vi "Move.vi"(8 "error in (no error)":errorcluster caption="错误输入（无错误）", 10 "samples per channel":i32=1000 caption="脉冲数", 11 "Hardware Resources in":T1 caption="硬件资源输入") -> (0 "error out":errorcluster caption="错误输出", 3 "Hardware Resources out":T1 caption="硬件资源输出")   [LabVIEW 2015, in "Motor Control.lvlib"]
doc: "初始化硬件引用。"
uses:
  Motor Control.lvlib
  Hardware Configuration.ctl
  <vilib>/DAQmx/create/channels.llb/DAQmx Create Channel (CO-Pulse Generation-Frequency).vi
  <vilib>/DAQmx/configure/timing.llb/DAQmx Timing (Implicit).vi
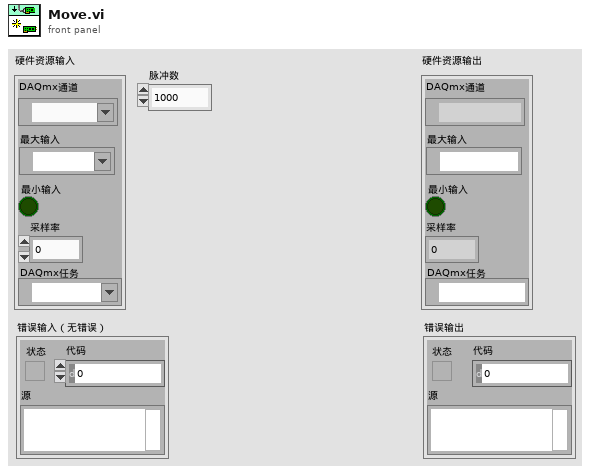
[diagram p1: front panel]
types:
  T1 = typedef "Motor Control.lvlib/Hardware Configuration.ctl" = cluster{"counter":tag, "方向端口":tag, "当前方向":bool, "频率":dbl, "DAQmx Task":refnum<k21>}
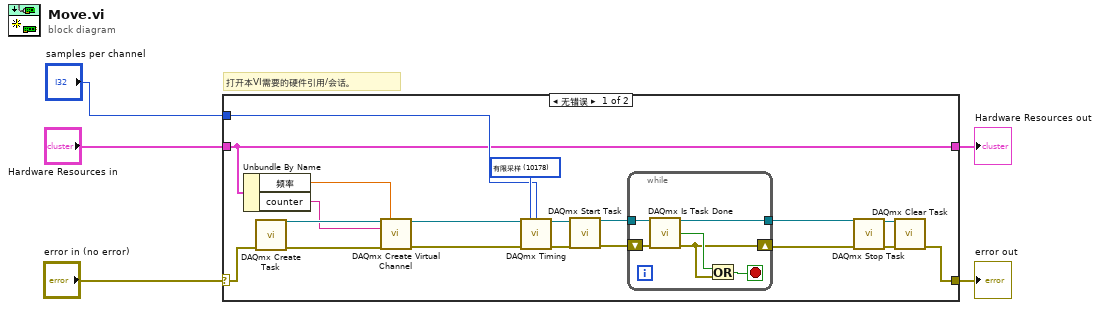
[diagram p0: block diagram]
diagram:
  # "打开本VI需要的硬件引用/会话。"
  n1 = case shown="无错误" "error in (no error)" {
    selector: "error in (no error)" -> [w20 w31]
    tunnel: [w19 w31] -> w4
    tunnel: "Hardware Resources in" -> [w12 w32]
    tunnel: [w12 w32] -> w2
    tunnel: "samples per channel" -> [w13 _]
    frame No Error {
      w14 = 10178 items=["有限采样"=10178, "连续采样"=10123, "硬件定时单点"=12522] ("sample mode")
      n2 = Unbundle By Name(w12) -> ("频率"=w17:dbl, "counter"=w18:tag)
      n3 = call <vilib>:"DAQmx Create Task.vi"("error in"=w20) -> ("task out"=w23:refnum<k21>, "error out"=w24:errorcluster)  [unwired: 13 in]
      n4 = call-poly <vilib>:"DAQmx Create Virtual Channel.vi"("task in"=w23, "frequency"=w17, "counter"=w18, "error in"=w24) -> ("task out"=w16:refnum<k21>, "error out"=w15:errorcluster)  [unwired: 10 in]
      n5 = call-poly <vilib>:"DAQmx Timing.vi"("task/channels in"=w16, "sample mode"=w14, "samples per channel"=w13, "error in"=w15) -> ("task out"=w11:refnum<k21>, "error out"=w10:errorcluster)  [unwired: 10 in]
      n6 = call <vilib>:"DAQmx Start Task.vi"("task/channels in"=w11, "error in"=w10) -> ("task out"=w9:refnum<k21>, "error out"=w8:errorcluster)  [unwired: 12 in]
      n7 = while {
        tunnel: w9 -> [w30]
        shift-right: [w26] -> w6
        shift-left: w8 -> [w29]
        tunnel: [w25] -> w7
        stop <- w27 stop-if-true
        n8 = call <vilib>:"DAQmx Is Task Done.vi"("task/channels in"=w30, "error in"=w29) -> ("task out"=w25:refnum<k21>, "task done?"=w28:bool, "error out"=w26:errorcluster)  [unwired: 11 in]
        n9 = Or(x=w28, y=w26) -> (x .or. y?=w27:bool)
      }
      n10 = call <vilib>:"DAQmx Stop Task.vi"("task/channels in"=w7, "error in"=w6) -> ("task out"=w21:refnum<k21>, "error out"=w22:errorcluster)  [unwired: 12 in]
      n11 = call <vilib>:"DAQmx Clear Task.vi"("task in"=w21, "error in"=w22) -> ("error out"=w19:errorcluster)  [unwired: 13 in]
    }
    frame Error {
    }
  }
  "Hardware Resources out" <- w2
  "error out" <- w4
